vi "20200930 sensor position theta measurment data_storage.vi"() -> ()   [LabVIEW 2016]
panel:
  in  "default value from gantry : X-Y-phi":dbl[](array[numeric])=[310.657, 1102.92, 0.011805]
  out "y pos Standard Dev 3":dbl
  out "y pos RMS 3":dbl
  out "y pos Arithmetic Mean 3":dbl
  out "phi pos Standard Dev 2":dbl
  out "phi pos RMS 2":dbl
  out "phi pos Arithmetic Mean 2":dbl
  out "x pos Standard Dev":dbl
  out "X pos RMS":dbl
  out "x pos Arithmetic Mean":dbl
  out "x pos":dbl[](array[numeric])
  out "y position":dbl[](array[numeric])
  out "phi":dbl[](array[numeric])
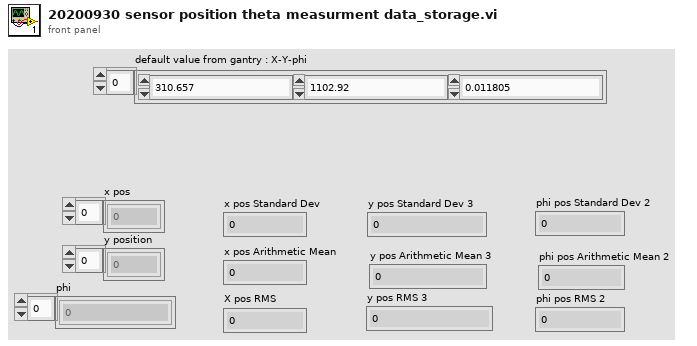
[diagram p1: front panel]
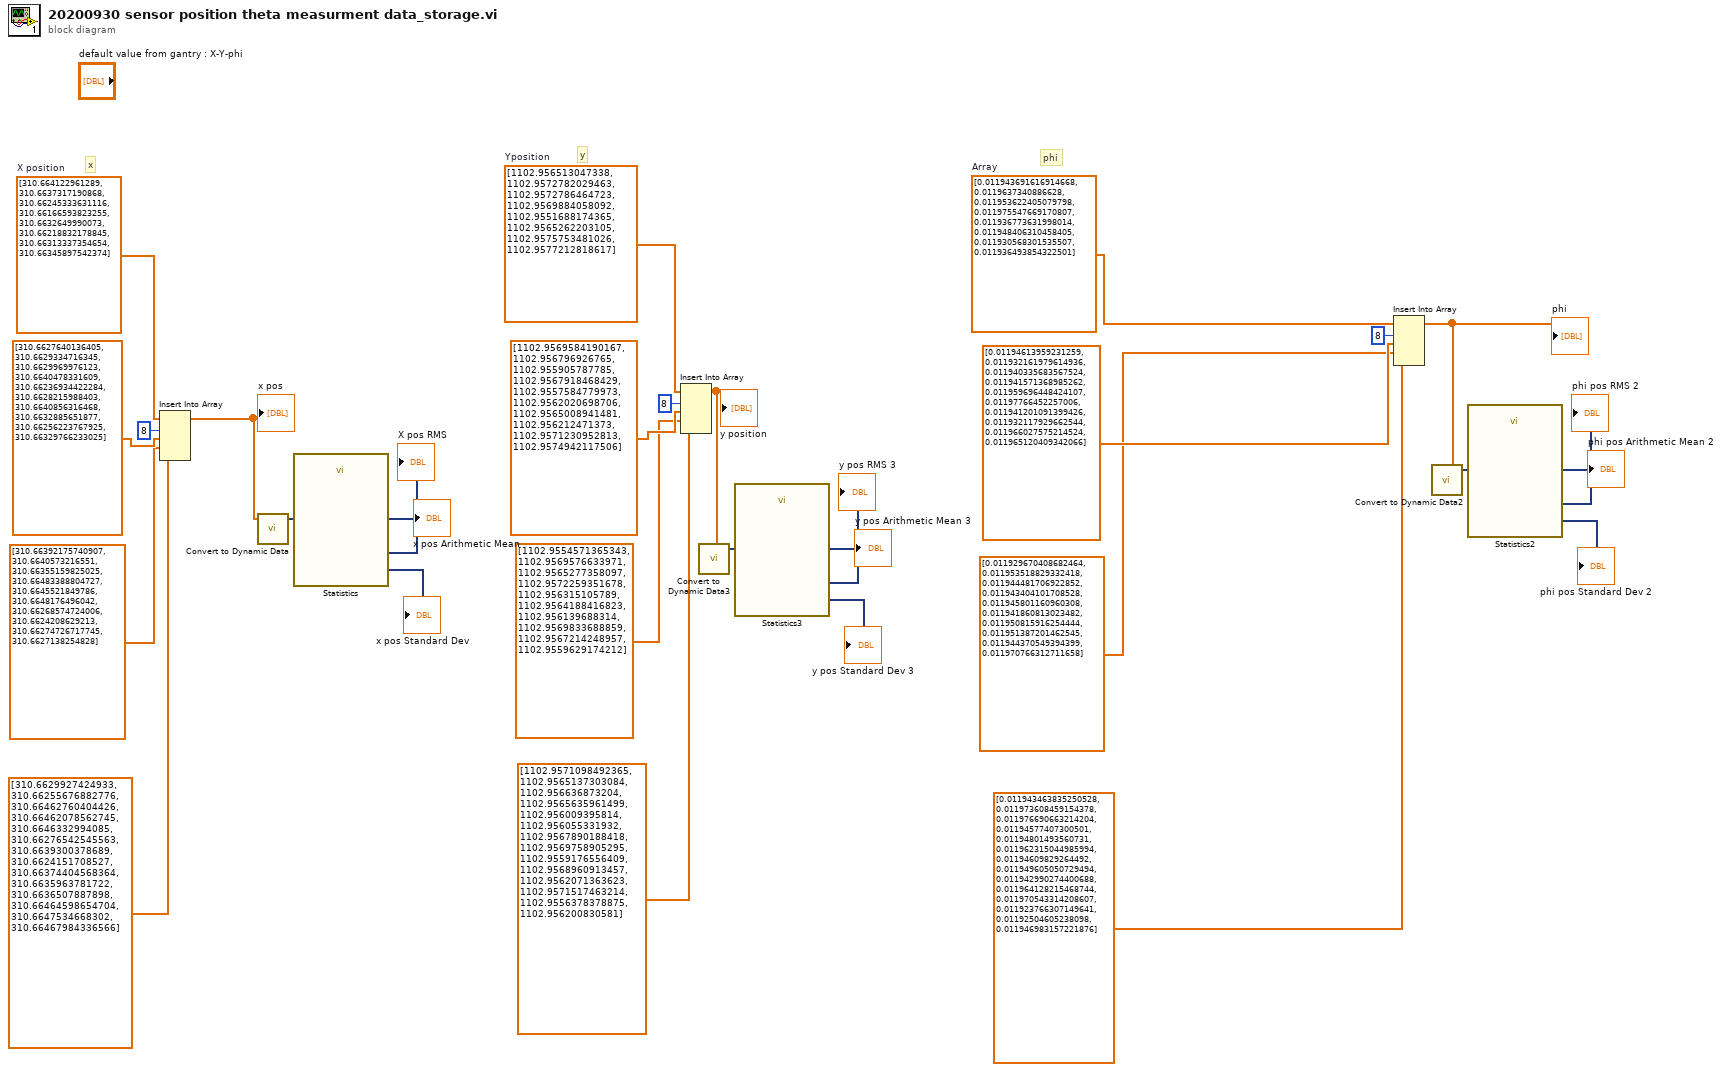
[diagram p0: block diagram]
diagram:
  w19 = dbl[] [310.664122961289, 310.6637317190868, 310.66245333631116, 310.66166593823255, 310.6632649990073, 310.66218832178845, 310.66313337354654, 310.66345897542374]  # X position
  w24 = dbl[] [1102.956513047338, 1102.9572782029463, 1102.9572786464723, 1102.9569884058092, 1102.9551688174365, 1102.9565262203105, 1102.9575753481026, 1102.9577212818617]  # Yposition
  w30 = dbl[] [0.011943691616914668, 0.0119637340886628, 0.011953622405079798, 0.011975547669170807, 0.011936773631998014, 0.011948406310458405, 0.011930568301535507, 0.011936493854322501]  # Array
  # "x"
  # "y"
  # "phi"
  n1 = Insert Into Array(array=w19, index=8, new element #1=dbl[] [310.6627640136405, 310.6629334716345, 310.6629969976123, 310.6640478331609, 310.66236934422284, 310.6628215988403, 310.6640856316468, 310.6632885651877, 310.66256223767925, 310.66329766233025] ("X position"), new element #2=dbl[] [310.66392175740907, 310.6640573216551, 310.66355159825025, 310.66483388804727, 310.6645521849786, 310.6648176496042, 310.66268574724006, 310.6624208629213, 310.66274726717745, 310.6627138254828] ("X position"), new element #3=dbl[] [310.6629927424933, 310.66255676882776, 310.66462760404426, 310.66462078562745, 310.6646332994085, 310.66276542545563, 310.6639300378689, 310.6624151708527, 310.66374404568364, 310.6635963781722, 310.6636507887898, 310.66464598654704, 310.6647534668302, 310.66467984336566] ("X position")) -> (w15:dbl[])
  "x pos" <- w15
  n2 = call "Convert to Dynamic Data"("Array"=w15) -> ("Dynamic Data Type"=w14:dynamicdata)  [unwired: 3 in]
  n3 = call "Statistics"("Signals"=w14) -> ("Standard Dev"=→"x pos Standard Dev":dynamicdata, "RMS"=→"X pos RMS":dynamicdata, "Arithmetic Mean"=→"x pos Arithmetic Mean":dynamicdata)  [unwired: 23 in, 1 out]
  n4 = Insert Into Array(array=w24, index=8, new element #1=dbl[] [1102.9569584190167, 1102.956796926765, 1102.955905787785, 1102.9567918468429, 1102.9557584779973, 1102.9562020698706, 1102.9565008941481, 1102.956212471373, 1102.9571230952813, 1102.9574942117506] ("Yposition"), new element #2=dbl[] [1102.9554571365343, 1102.9569576633971, 1102.9565277358097, 1102.9572259351678, 1102.956315105789, 1102.9564188416823, 1102.956139688314, 1102.9569833688859, 1102.9567214248957, 1102.9559629174212] ("Yposition"), new element #3=dbl[] [1102.9571098492365, 1102.9565137303084, 1102.956636873204, 1102.9565635961499, 1102.956009395814, 1102.956055331932, 1102.9567890188418, 1102.9569758905295, 1102.9559176556409, 1102.9568960913457, 1102.9562071363623, 1102.9571517463214, 1102.9556378378875, 1102.956200830581] ("Yposition")) -> (w2:dbl[])
  "y position" <- w2
  n5 = call "Convert to Dynamic Data3"("Array"=w2) -> ("Dynamic Data Type"=w1:dynamicdata)  [unwired: 3 in]
  n6 = call "Statistics3"("Signals"=w1) -> ("Standard Dev"=→"y pos Standard Dev 3":dynamicdata, "RMS"=→"y pos RMS 3":dynamicdata, "Arithmetic Mean"=→"y pos Arithmetic Mean 3":dynamicdata)  [unwired: 23 in, 1 out]
  n7 = Insert Into Array(array=w30, index=8, new element #1=dbl[] [0.01194613959231259, 0.011932161979614936, 0.011940335683567524, 0.011941571368985262, 0.011959696448424107, 0.01197766452257006, 0.011941201091399426, 0.011932117929662544, 0.011966027575214524, 0.011965120409342066] ("Array"), new element #2=dbl[] [0.011929670408682464, 0.011953518829332418, 0.011944481706922852, 0.011943404101708528, 0.011945801160960308, 0.011941860813023482, 0.011950815916254444, 0.011951387201462545, 0.011944370549394399, 0.011970766312711658] ("Array"), new element #3=dbl[] [0.011943463835250528, 0.011973608459154378, 0.011976690663214204, 0.01194577407300501, 0.01194801493560731, 0.011962315044985994, 0.01194609829264492, 0.011949605050729494, 0.011942990274400688, 0.011964128215468744, 0.011970543314208607, 0.011923766307149641, 0.01192504605238098, 0.011946983157221876] ("Array")) -> (w7:dbl[])
  "phi" <- w7
  n8 = call "Convert to Dynamic Data2"("Array"=w7) -> ("Dynamic Data Type"=w6:dynamicdata)  [unwired: 3 in]
  n9 = call "Statistics2"("Signals"=w6) -> ("Standard Dev"=→"phi pos Standard Dev 2":dynamicdata, "RMS"=→"phi pos RMS 2":dynamicdata, "Arithmetic Mean"=→"phi pos Arithmetic Mean 2":dynamicdata)  [unwired: 23 in, 1 out]
